vi "PXI-Launch Server.vi"(8 "error in (no error)":errorcluster) -> (0 "error out":errorcluster, 1 "Launched?":bool)   [LabVIEW 2020]
uses:
  Type Defs/Hardware Destination.ctl
  SGDA VIs/SGDA-Globals.vi
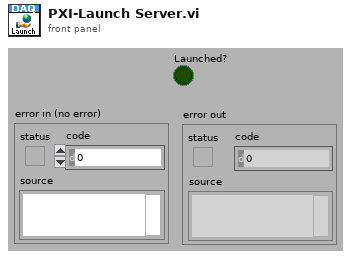
[diagram p1: front panel]
types:
  T1 = enum32{"Invalid", "Standard", "Closed", "Hidden", "Minimized", "Maximized"}
  T2 = typedef "Hardware Destination.ctl" = enum16{"None", "PXI", "TDT", "NI", "TDTSIM"}
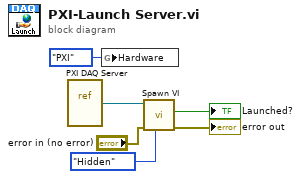
[diagram p0: block diagram]
diagram:
  n1 = vi-ref "PXI DAQ Server.vi"() -> (w5:refnum<vi>)
  n2 = global write "SGDA-Globals.vi" "Hardware"(Hardware_Destination."PXI" ("Hardware")) -> ()
  n3 = call "Spawn VI.vi"("State"=T1."Hidden", "error in (no error)"="error in (no error)", "VI reference"=w5) -> ("error out"=→"error out":errorcluster, "Started?"=→"Launched?":bool)  [unwired: 7 in]
